vi "Write Starting Timer Rate.vi"(8 "error in (no error)":errorcluster, 10 "Starting Timer Rate":i32=1000, 11 "Timing Engine in":refnum<class "Timing Engine.lvclass">) -> (0 "error out":errorcluster, 3 "Timing Engine out":refnum<class "Timing Engine.lvclass">)   [LabVIEW 2017, in "Assert API Components.lvlib" / "Assert Display.lvlib" / "Timing Engine.lvlib" / "Timing Engine.lvclass"]
uses:
  Timing Engine.lvclass
  Timing Engine.lvclass/Timing Engine.ctl
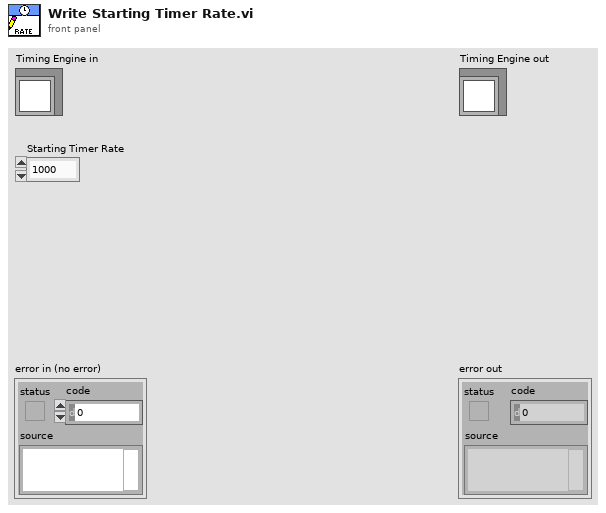
[diagram p1: front panel]
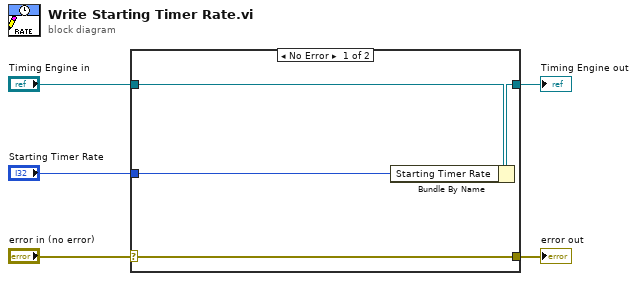
[diagram p0: block diagram]
diagram:
  n1 = case shown="No Error" "error in (no error)" {
    selector: "error in (no error)" -> [w9 w10]
    tunnel: [w9 w10] -> w4
    tunnel: [w7 w11] -> w2
    tunnel: "Timing Engine in" -> [w8 w11]
    tunnel: "Starting Timer Rate" -> [w6 _]
    frame No Error {
      n2 = Bundle By Name(cluster=w8, "Starting Timer Rate"=w6) -> (w7:refnum<class "Timing Engine.lvclass">)
    }
    frame Error {
    }
  }
  "error out" <- w4
  "Timing Engine out" <- w2
